vi "Periodic Tasks.vi"(8 "error in":errorcluster) -> ()   [LabVIEW 2018]
doc: "This VI runs in parallel to other tasks. It can contain as many user-defined periodic loops as you need. These can carry out PID or other sorts of timed response."
uses:
  <vilib>/Rock Robotics/WPI/ThirdParty/Phoenix-LabVIEW/Motor Controller/Controls/CTRE_Phoenix_MotorControl_ControlMode.ctl
  <vilib>/Rock Robotics/Network Tables/NT Read Numeric Array.vi
  <vilib>/Rock Robotics/Network Tables/NT Write Numeric Array.vi
panel:
  in  "Hatch motor power":dbl
  out "Hatch encoder":dbl
  in  "Angles":dbl(slide) scale=0.0..360.0
  in  "Motor power":dbl[](array[numeric])
  in  "Test type":T1(ring)
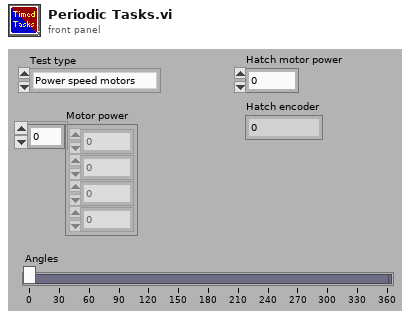
[diagram p1: front panel]
types:
  T1 = enum16{"Power speed motors", "Power angle motors", "Go to strafe angle", "Go to theta angles"}
  T2 = typedef "WPI_MotorControlDeviceRef.ctl" = cluster{"DeviceStatus":errorcluster, "Type":T3, "PWM":cluster{"PWM Channel":T4, "DeadBand":T5}, "CAN":cluster{"Device Number":u8, "SetOutput VI Ref":variant, "GetOutput VI Ref":variant, "Enable VI Ref":variant, "Disable VI Ref":variant, "Data":variant}, "Invert":bool, "DIO PWM":cluster{"PWM \"Enable\" Channel":T4, "DIOChannel":T6, "PWM Rate":dbl}}
  T3 = typedef "WPI_MotorControlType.ctl" = enum16{"PWM", "CAN", "DIO PWM"}
  T4 = typedef "FPGA_DIOPWMChannel.ctl" = enum8{"PWM 0", "PWM 1", "PWM 2", "PWM 3", "PWM 4", "PWM 5", "PWM 6", "PWM 7", "PWM 8", "PWM 9", "PWM MXP 0", "PWM MXP 1", "PWM MXP 2", "PWM MXP 3", "PWM MXP 4", "PWM MXP 5", "PWM MXP 6", "PWM MXP 7", "PWM MXP 8", "PWM MXP 9", "Invalid"}
  T5 = typedef "WPI_PWMDeadband.ctl" = cluster{"Name":string, "maxPositivePwm":i32, "minPositivePwm":i32, "centerPwm":i32, "maxNegativePwm":i32, "minNegativePwm":i32, "angularRange":u16}
  T6 = typedef "FPGA_DIOChannel.ctl" = enum8{"DIO 0", "DIO 1", "DIO 2", "DIO 3", "DIO 4", "DIO 5", "DIO 6", "DIO 7", "DIO 8", "DIO 9", "DIO MXP 0", "DIO MXP 1", "DIO MXP 2", "DIO MXP 3", "DIO MXP 4", "DIO MXP 5", "DIO MXP 6", "DIO MXP 7", "DIO MXP 8", "DIO MXP 9", "DIO MXP 10", "DIO MXP 11", "DIO MXP 12", "DIO MXP 13", "DIO MXP 14", "DIO MXP 15", "SPI Port CS1", "SPI Port CS2", "SPI Port CS3", "SPI Port MISO", "SPI Port MOSI", "Invalid"}
  T7 = typedef "WPI_AnalogChannelDevRef.ctl" = cluster{"DevStatus":errorcluster, "Analog Channel":T8}
  T8 = typedef "FPGA_AIChannel.ctl" = enum8{"AI 0", "AI 1", "AI 2", "AI 3", "AI MXP 0", "AI MXP 1", "AI MXP 2", "AI MXP 3", "Invalid"}
  T9 = typedef "WPI_EncoderDevRef.ctl" = cluster{"DevStatus":errorcluster, "EncoderIndex":T10, "CounterIndex":T11, "DistancePerCount":dbl, "Decoding Type":T12}
  T10 = typedef "FPGA_EncoderIdx.ctl" = enum8{"Enc 0", "Enc 1", "Enc 2", "Enc 3", "Enc 4", "Enc 5", "Enc 6", "Enc 7", "Invalid"}
  T11 = typedef "FPGA_CounterCtrSystemIndex.ctl" = enum8{"Ctr 0", "Ctr 1", "Ctr 2", "Ctr 3", "Ctr 4", "Ctr 5", "Ctr 6", "Ctr 7", "Invalid"}
  T12 = typedef "WPI_EncoderType.ctl" = enum16{"1x", "2x", "4x"}
  T13 = cluster{"PhoenixMotorControlDevRef":T2, "PhoenixMotorControlDevRef":T2, "PhoenixMotorControlDevRef":T2, "PhoenixMotorControlDevRef":T2}
  T14 = typedef "CTRE_Phoenix_MotorControl_ControlMode.ctl" = u16
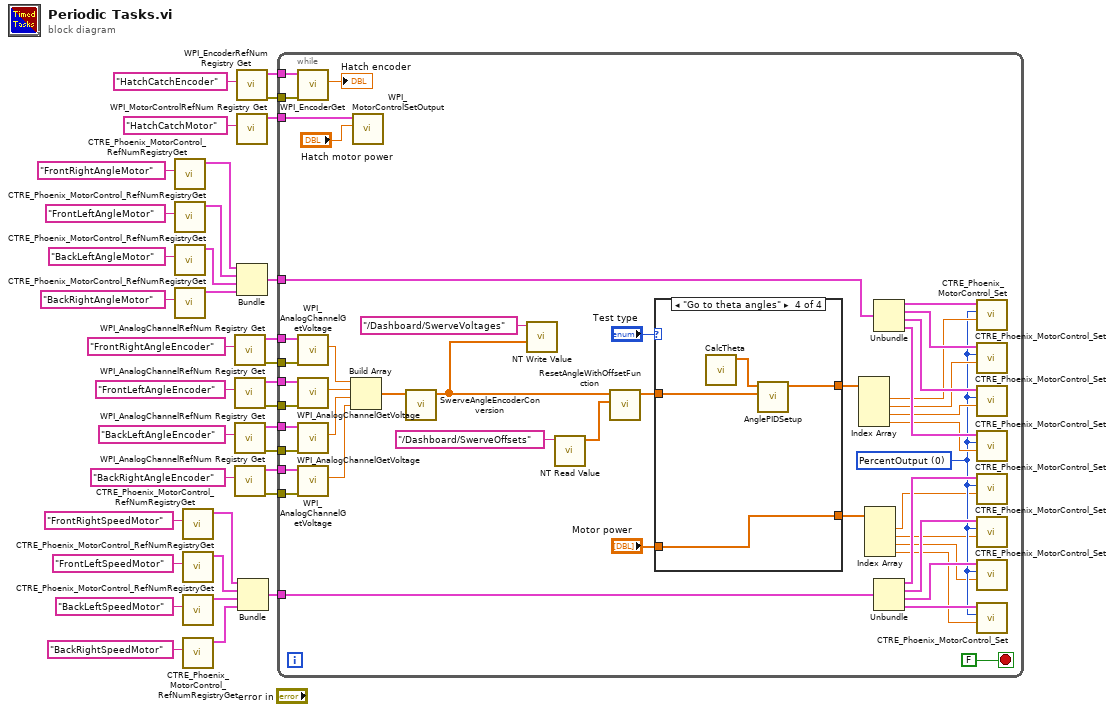
[diagram p0: block diagram]
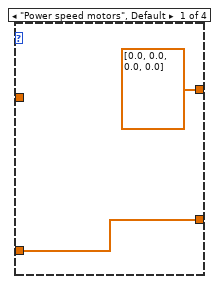
[diagram p2: hidden frame]
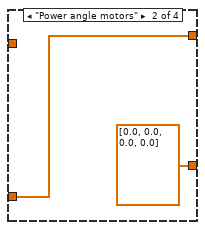
[diagram p3: hidden frame]
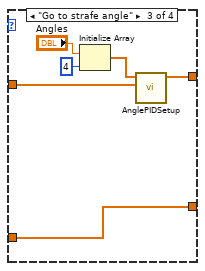
[diagram p4: hidden frame]
diagram:
  n1 = call <vilib>:"CTRE_Phoenix_MotorControl_RefNumRegistryGet.vi"("refnum name"="FrontRightAngleMotor") -> ("PhoenixMotorControlDevRef"=w15:T2)  [unwired: 9 in, 1 out]
  n2 = call <vilib>:"CTRE_Phoenix_MotorControl_RefNumRegistryGet.vi"("refnum name"="FrontLeftAngleMotor") -> ("PhoenixMotorControlDevRef"=w14:T2)  [unwired: 9 in, 1 out]
  n3 = call <vilib>:"CTRE_Phoenix_MotorControl_RefNumRegistryGet.vi"("refnum name"="BackLeftAngleMotor") -> ("PhoenixMotorControlDevRef"=w13:T2)  [unwired: 9 in, 1 out]
  n4 = call <vilib>:"CTRE_Phoenix_MotorControl_RefNumRegistryGet.vi"("refnum name"="BackRightAngleMotor") -> ("PhoenixMotorControlDevRef"=w12:T2)  [unwired: 9 in, 1 out]
  n5 = call <vilib>:"CTRE_Phoenix_MotorControl_RefNumRegistryGet.vi"("refnum name"="FrontRightSpeedMotor") -> ("PhoenixMotorControlDevRef"=w6:T2)  [unwired: 9 in, 1 out]
  n6 = call <vilib>:"CTRE_Phoenix_MotorControl_RefNumRegistryGet.vi"("refnum name"="FrontLeftSpeedMotor") -> ("PhoenixMotorControlDevRef"=w7:T2)  [unwired: 9 in, 1 out]
  n7 = call <vilib>:"CTRE_Phoenix_MotorControl_RefNumRegistryGet.vi"("refnum name"="BackLeftSpeedMotor") -> ("PhoenixMotorControlDevRef"=w8:T2)  [unwired: 9 in, 1 out]
  n8 = call <vilib>:"CTRE_Phoenix_MotorControl_RefNumRegistryGet.vi"("refnum name"="BackRightSpeedMotor") -> ("PhoenixMotorControlDevRef"=w9:T2)  [unwired: 9 in, 1 out]
  n9 = call <vilib>:"WPI_AnalogChannelRefNum Registry Get.vi"("refnum name"="FrontRightAngleEncoder") -> ("error out"=w23:errorcluster, "AIDeviceRef"=w22:T7)  [unwired: 9 in]
  n10 = call <vilib>:"WPI_AnalogChannelRefNum Registry Get.vi"("refnum name"="FrontLeftAngleEncoder") -> ("error out"=w20:errorcluster, "AIDeviceRef"=w21:T7)  [unwired: 9 in]
  n11 = call <vilib>:"WPI_AnalogChannelRefNum Registry Get.vi"("refnum name"="BackLeftAngleEncoder") -> ("error out"=w18:errorcluster, "AIDeviceRef"=w19:T7)  [unwired: 9 in]
  n12 = call <vilib>:"WPI_AnalogChannelRefNum Registry Get.vi"("refnum name"="BackRightAngleEncoder") -> ("error out"=w16:errorcluster, "AIDeviceRef"=w17:T7)  [unwired: 9 in]
  n13 = call <vilib>:"WPI_EncoderRefNum Registry Get.vi"("refnum name"="HatchCatchEncoder") -> ("error out"=w1:errorcluster, "EncoderDevRef"=w2:T9)  [unwired: 9 in]
  n14 = call <vilib>:"WPI_MotorControlRefNum Registry Get.vi"("refnum name"="HatchCatchMotor") -> ("MotorControlDevRef"=w3:T2)  [unwired: 9 in, 1 out]
  n15 = Bundle("PhoenixMotorControlDevRef"=w15, "PhoenixMotorControlDevRef"=w14, "PhoenixMotorControlDevRef"=w13, "PhoenixMotorControlDevRef"=w12) -> (w11:T13)  [unwired: 1 in]
  n16 = Bundle("PhoenixMotorControlDevRef"=w6, "PhoenixMotorControlDevRef"=w7, "PhoenixMotorControlDevRef"=w8, "PhoenixMotorControlDevRef"=w9) -> (w10:T13)  [unwired: 1 in]
  n17 = while {
    tunnel: w23 -> [w79]
    tunnel: w22 -> [w78]
    tunnel: w21 -> [w77]
    tunnel: w20 -> [w76]
    tunnel: w19 -> [w75]
    tunnel: w18 -> [w74]
    tunnel: w17 -> [w73]
    tunnel: w16 -> [w72]
    tunnel: w11 -> [w65]
    tunnel: w10 -> [w66]
    tunnel: w3 -> [w50]
    tunnel: w2 -> [w49]
    tunnel: w1 -> [w48]
    stop <- FALSE stop-if-true
    w45 = T14 0 items=["PercentOutput"=0, "Position"=1, "Velocity"=2, "Current"=3, "Follower"=5, "MotionProfile"=6, "MotionMagic"=7, "MotionProfileArc"=10, "Disabled"=15] ("Control Mode")
    n18 = call <vilib>:"WPI_EncoderGet.vi"("error in (no error)"=w48, "EncoderDevRef"=w49) -> ("Distance"=→"Hatch encoder":dbl)  [unwired: 4 in, 5 out]
    n19 = call <vilib>:"WPI_AnalogChannelGetVoltage.vi"("error in (no error)"=w79, "AIDeviceRef"=w78) -> ("Voltage"=w62:dbl)  [unwired: 7 in, 2 out]
    n20 = call <vilib>:"WPI_AnalogChannelGetVoltage.vi"("error in (no error)"=w76, "AIDeviceRef"=w77) -> ("Voltage"=w61:dbl)  [unwired: 7 in, 2 out]
    n21 = call <vilib>:"WPI_AnalogChannelGetVoltage.vi"("error in (no error)"=w74, "AIDeviceRef"=w75) -> ("Voltage"=w60:dbl)  [unwired: 7 in, 2 out]
    n22 = call <vilib>:"WPI_AnalogChannelGetVoltage.vi"("error in (no error)"=w72, "AIDeviceRef"=w73) -> ("Voltage"=w59:dbl)  [unwired: 7 in, 2 out]
    n23 = Build Array(w62, w61, w60, w59) -> (w39:dbl[])
    n24 = call <vilib>:"WPI_MotorControlSetOutput.vi"("Output"="Hatch motor power", "MotorControlDevRef"=w50) -> ()  [unwired: 7 in, 3 out]
    n25 = call "SwerveAngleEncoderConversion.vi"("Voltages"=w39) -> ("Angles"=w37:dbl[])  [unwired: 10 in]
    n26 = call-poly <vilib>:"NT Write Value.vi"("Numeric Array"=w37, "Name"="/Dashboard/SwerveVoltages") -> ()  [unwired: 9 in, 1 out]
    n27 = call-poly <vilib>:"NT Read Value.vi"("Name"="/Dashboard/SwerveOffsets") -> ("Numeric Array"=w36:dbl[])  [unwired: 9 in, 1 out]
    n28 = call "ResetAngleWithOffsetFunction.vi"("Offset"=w36, "AngleInput"=w37) -> ("AngleOutput"=w38:dbl[])  [unwired: 9 in]
    n29 = case shown="\"Go to theta angles\"" "Test type" {
      tunnel: "Motor power" -> [w84 w86 w87 w96]
      tunnel: [w84 dbl[] [0.0, 0.0, 0.0, 0.0] ("Motor power") w87 w96] -> w44
      tunnel: [dbl[] [0.0, 0.0, 0.0, 0.0] ("Output") w86 w91 w94] -> w55
      tunnel: w38 -> [_ _ w92 w93]
      frame "Power speed motors", Default {
      }
      frame "Power angle motors" {
      }
      frame "Go to strafe angle" {
        n30 = Initialize Array("Angles", 4 ("dimension size")) -> (w88:dbl[])
        n31 = call "AnglePIDSetup.vi"("Encoder"=w92, "Setpoint"=w88) -> ("Output"=w91:dbl[])  [unwired: 9 in]
      }
      frame "Go to theta angles" {
        n32 = call "CalcTheta.vi"() -> ("ThetaValues"=w95:dbl[])  [unwired: 11 in]
        n33 = call "AnglePIDSetup.vi"("Encoder"=w93, "Setpoint"=w95) -> ("Output"=w94:dbl[])  [unwired: 9 in]
      }
    }
    n34 = Index Array(array=w55) -> (element #1=w54:dbl, element #2=w53:dbl, element #3=w52:dbl, element #4=w51:dbl)  [unwired: 4 in]
    n35 = Index Array(array=w44) -> (element #1=w43:dbl, element #2=w42:dbl, element #3=w40:dbl, element #4=w41:dbl)  [unwired: 4 in]
    n36 = Unbundle(w65) -> ("PhoenixMotorControlDevRef"=w71:T2, "PhoenixMotorControlDevRef"=w70:T2, "PhoenixMotorControlDevRef"=w69:T2, "PhoenixMotorControlDevRef"=w68:T2)
    n37 = Unbundle(w66) -> ("PhoenixMotorControlDevRef"=w56:T2, "PhoenixMotorControlDevRef"=w64:T2, "PhoenixMotorControlDevRef"=w63:T2, "PhoenixMotorControlDevRef"=w67:T2)
    n38 = call <vilib>:"CTRE_Phoenix_MotorControl_Set.vi"("Output"=w54, "Control Mode"=w45, "PhoenixMotorControlDevRef"=w71) -> ()  [unwired: 7 in, 2 out]
    n39 = call <vilib>:"CTRE_Phoenix_MotorControl_Set.vi"("Output"=w53, "Control Mode"=w45, "PhoenixMotorControlDevRef"=w70) -> ()  [unwired: 7 in, 2 out]
    n40 = call <vilib>:"CTRE_Phoenix_MotorControl_Set.vi"("Output"=w52, "Control Mode"=w45, "PhoenixMotorControlDevRef"=w69) -> ()  [unwired: 7 in, 2 out]
    n41 = call <vilib>:"CTRE_Phoenix_MotorControl_Set.vi"("Output"=w51, "Control Mode"=w45, "PhoenixMotorControlDevRef"=w68) -> ()  [unwired: 7 in, 2 out]
    n42 = call <vilib>:"CTRE_Phoenix_MotorControl_Set.vi"("Output"=w43, "Control Mode"=w45, "PhoenixMotorControlDevRef"=w56) -> ()  [unwired: 7 in, 2 out]
    n43 = call <vilib>:"CTRE_Phoenix_MotorControl_Set.vi"("Output"=w42, "Control Mode"=w45, "PhoenixMotorControlDevRef"=w64) -> ()  [unwired: 7 in, 2 out]
    n44 = call <vilib>:"CTRE_Phoenix_MotorControl_Set.vi"("Output"=w40, "Control Mode"=w45, "PhoenixMotorControlDevRef"=w63) -> ()  [unwired: 7 in, 2 out]
    n45 = call <vilib>:"CTRE_Phoenix_MotorControl_Set.vi"("Output"=w41, "Control Mode"=w45, "PhoenixMotorControlDevRef"=w67) -> ()  [unwired: 7 in, 2 out]
  }
